vi "Omni-Bus Inject CSGL.vi"(6 "Enable":bool, 8 "error in (no error)":errorcluster, 9 "Injected Value":csg, 10 "Tag":string, 11 "Omni_Bus in":refnum<class "Omni_Bus.lvclass">) -> (0 "error out":errorcluster, 3 "Omni_Bus out":refnum<class "Omni_Bus.lvclass">)   [LabVIEW 2021, in "Fault-Injection Bus.lvclass"]
uses:
  Fault-Injection Bus.lvclass
  Omni-Bus/Omni_Bus.lvclass
  Value Type/CSGL/Fault-Injection_CSGL.lvclass
  C:/Program Files (x86)/National Instruments/LabVIEW 2021/vi.lib/TSA/Abstract Data Classes/Abs_Types/Type/Abs_Type.lvclass
  <vilib>/TSA/Abstract Data Classes/Abs_Types/Type/Abs_Type.lvclass/Abs_Type.ctl
  Omni-Bus/Omni_Bus.lvclass/Omni_Bus.ctl
  <vilib>/Utility/error.llb/Clear Errors.vi
  Omni-Bus/Properties/Read Var Map.vi
  <vilib>/TSA/Abstract Data Classes/Abs_Types/Type/Properties/Read Tag.vi
  <vilib>/TSA/Abstract Data Classes/Abs_Types/Value/Abs_Value.lvclass
  Omni-Bus/Support/Check For Read Only Error.vi
  Omni-Bus/Support/Incorrect Tag String Error.vi
  <vilib>/TSA/Abstract Data Classes/Abs_Types/Type/Abs_Type.lvclass
  Fault-Injection Bus.lvclass/Fault-Injection Bus.ctl
  C:/Program Files (x86)/National Instruments/LabVIEW 2021/vi.lib/TSA/Abstract Data Classes/Abs_Types/Complex Single Float/Abs_Complex Single Float.lvclass
  C:/Program Files (x86)/National Instruments/LabVIEW 2021/vi.lib/TSA/Abstract Data Classes/Abs_Types/Floating Point/Abs_Floating Point.lvclass
  C:/Program Files (x86)/National Instruments/LabVIEW 2021/vi.lib/TSA/Abstract Data Classes/Abs_Types/Numeric/Abs_Numeric.lvclass
  C:/Program Files (x86)/National Instruments/LabVIEW 2021/vi.lib/TSA/Abstract Data Classes/Abs_Types/Value/Abs_Value.lvclass
  C:/TSA/Omni-Bus/Source/Fault-Injection Bus/Support/Interfaces/CSGL/Fault-Injection_CSGL_Type.lvclass
  C:/TSA/Omni-Bus/Source/Fault-Injection Bus/Support/Interfaces/Type/Fault-Injection_Type.lvclass
  C:/TSA/Omni-Bus/Source/Fault-Injection Bus/Support/Value Type/CSGL/Fault-Injection_CSGL.lvclass
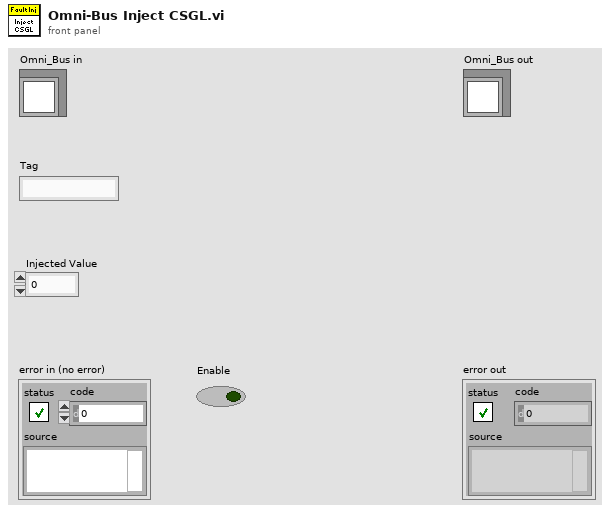
[diagram p1: front panel]
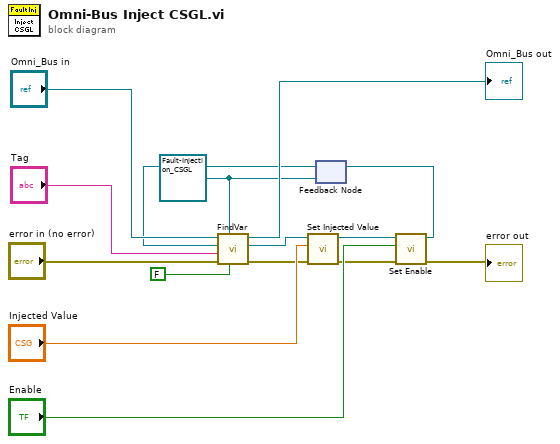
[diagram p0: block diagram]
diagram:
  w1 = refnum<class "Fault-Injection_CSGL.lvclass"> refnum ("Fault-Injection_Boolean out")
  n1 = feedback #1(w1) -> (w6:refnum<class "Fault-Injection_CSGL.lvclass">)
  n2 = call "FindVar.vi"("Write?"=FALSE, "Abs_Type"=w1, "error in (no error)"="error in (no error)", "Tag"="Tag", "Abs_Type Default"=w6, "Var Bus in"="Omni_Bus in") -> ("error out"=w8:errorcluster, "Abs_Type Found"=w7:refnum<class "Fault-Injection_CSGL.lvclass">, "Var Bus out"=→"Omni_Bus out":refnum<class "Omni_Bus.lvclass">)  [unwired: 2 in, 1 out]
  n3 = call-dynamic "Set Injected Value.vi"("error in (no error)"=w8, "Value"="Injected Value", "Fault-Injection_Boolean in"=w7) -> ("error out"=w5:errorcluster, "Fault-Injection_Boolean out"=w4:refnum<class "Fault-Injection_CSGL.lvclass">)  [unwired: 7 in]
  n4 = call-dynamic "Set Enable.vi"("error in (no error)"=w5, "Enable"="Enable", "Fault-Injection_Boolean in"=w4) -> ("error out"=→"error out":errorcluster, "Fault-Injection_Boolean out"=w3:refnum<class "Fault-Injection_CSGL.lvclass">)  [unwired: 7 in]
  n5 = feedback-in #1(w3) -> ()
